vi "Request_DO_DI.vi"(8 "error in (no error)":errorcluster, 9 "quantity":u16, 10 "starting address":u16) -> (0 "error out":errorcluster, 2 "MB_PDU":T1={"Function Code"=1, "Data"=[], "RTU_DataBytes"=0})   [LabVIEW 2016]
uses:
  MB_PDU/MB_PDU_Cluster.ctl
  MB Master.lvlib
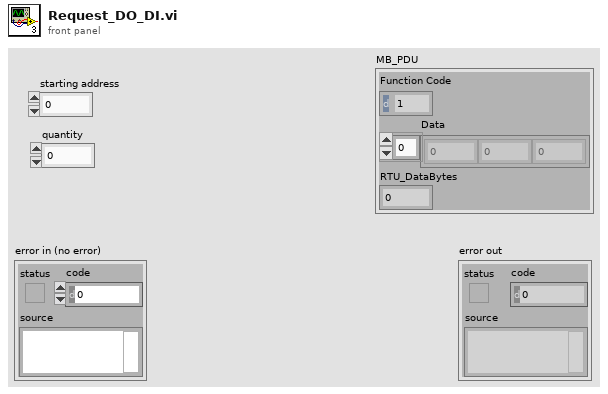
[diagram p1: front panel]
types:
  T1 = typedef "MB Master.lvlib/MB_PDU_Cluster.ctl" = cluster{"Function Code":u8, "Data":u8[], "RTU_DataBytes":i32}
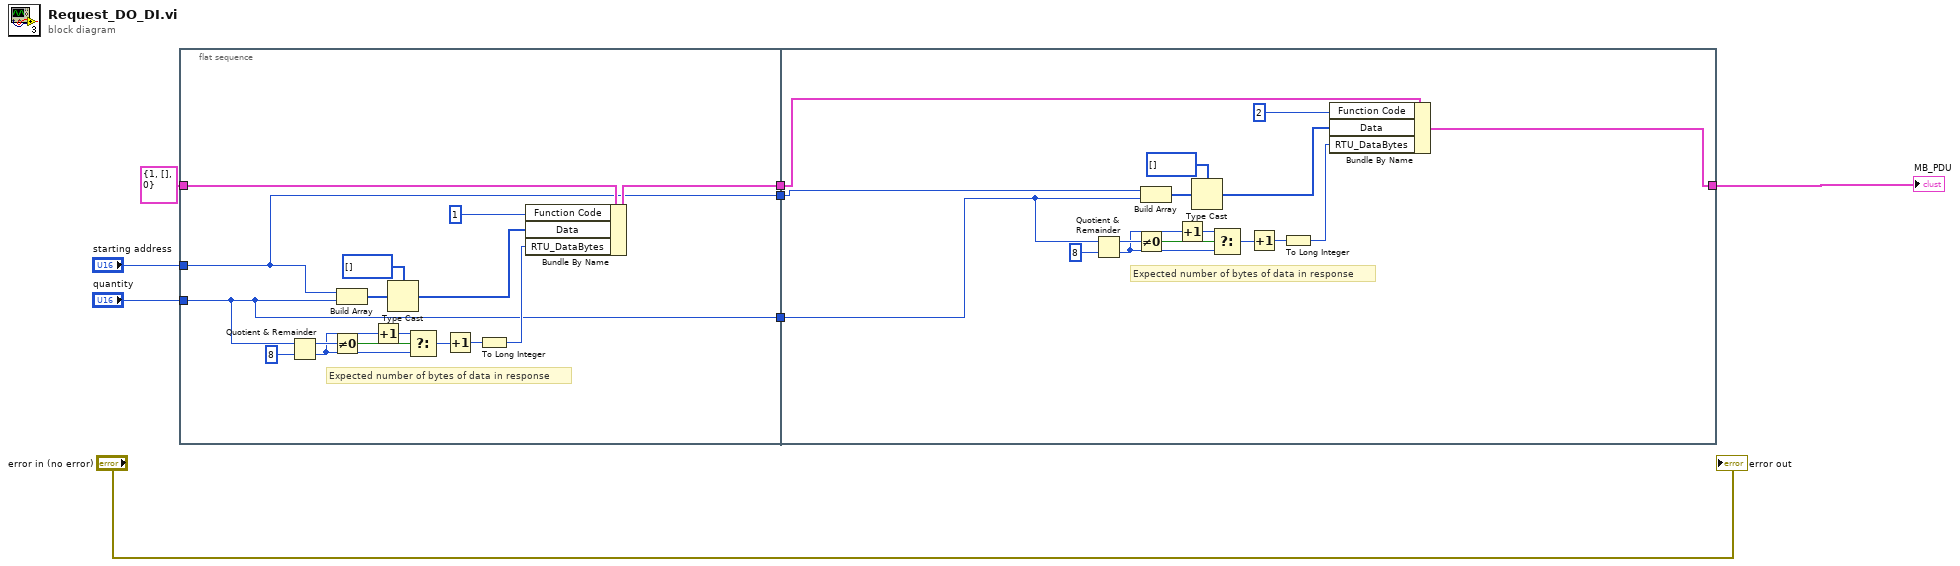
[diagram p0: block diagram]
diagram:
  n1 = flat-sequence {
    tunnel: "starting address" -> [w10]
    tunnel: T1 {"Function Code"=1, "Data"=[], "RTU_DataBytes"=0} ("Modbus Serial New.lvlib:MB_PDU.lvclass") -> [w22]
    tunnel: "quantity" -> [w9]
    tunnel: [w19] -> w3
    tunnel: [w10] -> w2
    tunnel: [w9] -> w1
    tunnel: [w27] -> w6
    tunnel: w3 -> [w28]
    tunnel: w2 -> [w26]
    tunnel: w1 -> [w25]
    frame #0 {
      # "Expected number of bytes of data in response"
      n2 = Quotient & Remainder(x=w9, y=u16 8) -> (x-y*floor(x/y)=w17:u16, floor(x/y)=w14:u16)
      n3 = Not Equal To 0?(x=w17) -> (x != 0?=w16:bool)
      n4 = Build Array(w10, w9) -> (w24:u16[])
      n5 = Increment(x=w14) -> (x+1=w15:u16)
      n6 = Type Cast(type=u8[] [], x=w24) -> (*(type *) &x=w20:u8[])
      n7 = Select(t=w15, s=w16, f=w14) -> (s? t:f=w12:u16)
      n8 = Increment(x=w12) -> (x+1=w11:u16)
      n9 = To Long Integer(number=w11) -> (32bit integer=w13:i32)
      n10 = Bundle By Name(cluster=w22, "Function Code"=u8 1, "Data"=w20, "RTU_DataBytes"=w13) -> (w19:T1)
    }
    frame #1 {
      # "Expected number of bytes of data in response"
      n11 = Quotient & Remainder(x=w25, y=u16 8) -> (x-y*floor(x/y)=w35:u16, floor(x/y)=w32:u16)
      n12 = Not Equal To 0?(x=w35) -> (x != 0?=w34:bool)
      n13 = Build Array(w26, w25) -> (w40:u16[])
      n14 = Increment(x=w32) -> (x+1=w33:u16)
      n15 = Type Cast(type=u8[] [], x=w40) -> (*(type *) &x=w37:u8[])
      n16 = Select(t=w33, s=w34, f=w32) -> (s? t:f=w30:u16)
      n17 = Increment(x=w30) -> (x+1=w29:u16)
      n18 = To Long Integer(number=w29) -> (32bit integer=w31:i32)
      n19 = Bundle By Name(cluster=w28, "Function Code"=u8 2, "Data"=w37, "RTU_DataBytes"=w31) -> (w27:T1)
    }
  }
  "error out" <- "error in (no error)"
  "MB_PDU" <- w6
